vi "UiCharts_gm.vi"() -> ()   [LabVIEW 2011]
uses:
  Output - Cluster gas.ctl
  DBSqlSelectToArray(2DArrayString).vi
panel:
  in  "Tab Control":T1(tab)
  out "protocol":string[][](table)
  out "Temperaturregelung":cluster{"GM TS-2[°C]":dbl}(graph)
  in  "load":bool
  out "XY Graph":cluster{timestamp, dbl}[](graph)
  in  "end":timestamp=timestamp(3427221599.999 s since 1904-01-01) format="%<%X\n%x>T"
  in  "begin":timestamp=timestamp(3427135200 s since 1904-01-01) format="%<%X\n%x>T"
  in  "sensor":u16(ring) items=["DS1"=0, "TS4"=2, "TS5"=4, "pHS1"=6, "FS1"=8, "FS2"=10, "FS3"=12]
  in  "plant":u16(ring)=1 items=["B2G1", "B2G2", "GasMeas"]
  out "error out":errorcluster
  in  "stop":bool
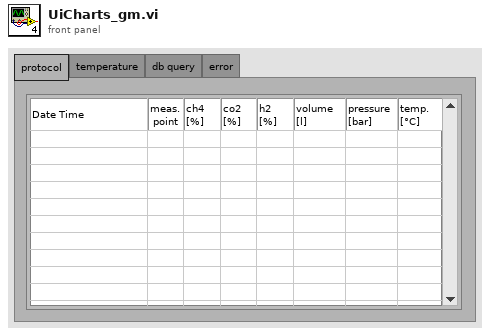
[diagram p1: front panel]
types:
  T1 = enum32{"protocol", "temperature", "db query", "error"}
  T2 = typedef "Output - Cluster gas.ctl" = cluster{"B2G2 MR V1.1 AUF":bool, "B2G2 MR V1.1 ZU":bool, "B2G2 MR V1 AUF":bool, "B2G2 MR V1 ZU":bool, "B2G1 T2 V1 AUF":bool, "B2G1 T2 V1 ZU":bool, "B2G1 T2 V1.1 AUF":bool, "B2G1 T2 V1.1 ZU":bool, "B2G2 T2 V1 AUF":bool, "B2G2 T2 V1 ZU":bool, "B2G2 T2 V1.1 ZU":bool, "B2G2 T2 V1.1 AUF":bool, "B2G1 MR V1 AUF":bool, "B2G1 MR V1 ZU":bool, "B2G1 MR V1.1 AUF":bool, "B2G1 MR V1.1 ZU":bool, "B2G1 HR V1 AUF":bool, "B2G1 HR V1 ZU":bool, "B2G1 HR V1.1 AUF":bool, "B2G1 HR V1.1 ZU":bool, "Fab1 HR V1 AUF":bool, "Fab1 HR V1 ZU":bool, "Fab1 HR V1.1 AUF":bool, "Fab1 HR V1.1 ZU":bool, "Fab1 MR V1 AUF":bool, "Fab1 MR V1 ZU":bool, "Fab1 MR V1.1 AUF":bool, "Fab1 MR V1.1 ZU":bool, "Fab1 BL V1 AUF":bool, "Fab1 BL V1 ZU":bool, "Fab1 BL V1.1 AUF":bool, "Fab1 BL V1.1 ZU":bool, "Fab2 HR V1 AUF":bool, "Fab2 HR V1 ZU":bool, "Fab2 HR V1.1 AUF":bool, "Fab2 HR V1.1 ZU":bool, "Fab2 MR V1 AUF":bool, "Fab2 MR V1 ZU":bool, "Fab2 MR V1.1 AUF":bool, "Fab2 MR V1.1 ZU":bool, "GA1 ch4 [%]":dbl, "GA1 co2 [%]":dbl, "GA1 h2 [%]":dbl, "GM P1 RUN":bool, "GM V-1 AUF":bool, "GM V-1 ZU":bool, "GM V-2 AUF":bool, "GM V-2 ZU":bool, "GM V-3 AUF":bool, "GM V-3 ZU":bool, "GM V-4 AUF":bool, "GM V-4 ZU":bool, "GM P2 RUN":bool, "GM GZ-1 [imp]":u32, "GM DS-2 [bar]":dbl, "GM DS-1 [bar]":dbl, "GM TS-1 [°C]":dbl, "GM TS-2[°C]":dbl, "gas_values":cluster{"timestamp":timestamp, "GM DS-2 [bar]":dbl, "GA1 ch4 [%]":dbl, "GA1 co2 [%]":dbl, "GA1 h2 [%]":dbl, "GM DS-1 [bar]":dbl, "GM TS-1 [°C]":dbl, "GM TS-2 [°C]":dbl, "GM GZ-1 [l]":dbl, "empty":bool, "measuring point":u8}, "measuring mode":u8}
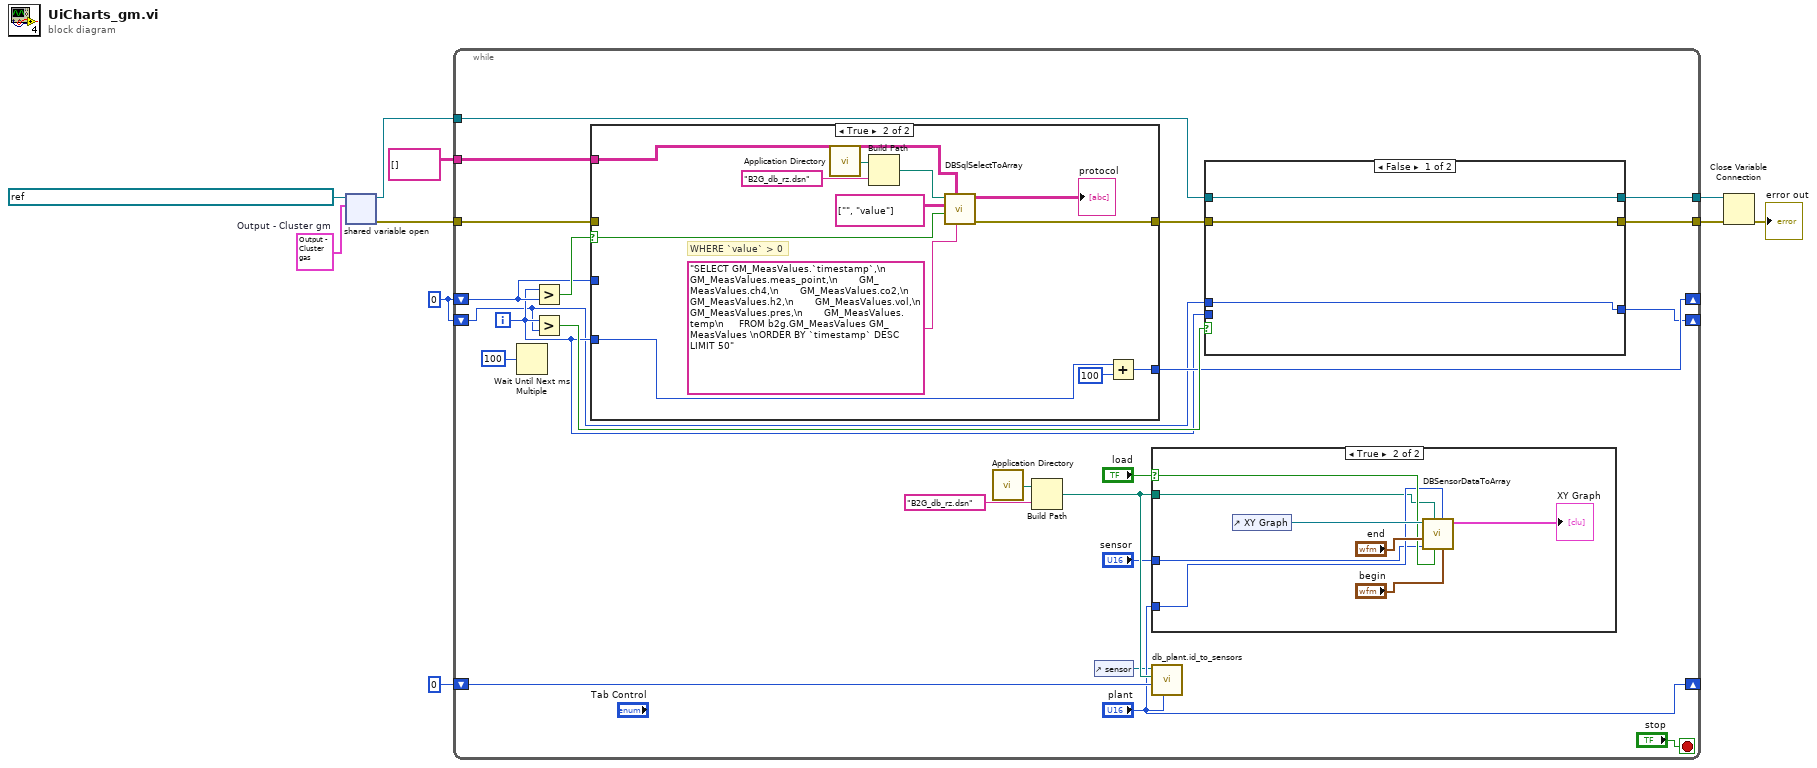
[diagram p0: block diagram]
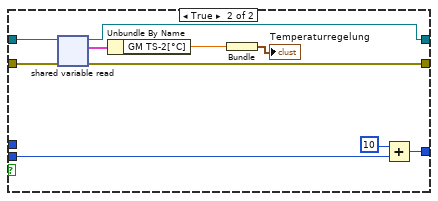
[diagram p4: hidden frame]
diagram:
  w9 = T2 {"B2G2 MR V1.1 AUF"=FALSE, "B2G2 MR V1.1 ZU"=FALSE, "B2G2 MR V1 AUF"=FALSE, "B2G2 MR V1 ZU"=FALSE, "B2G1 T2 V1 AUF"=FALSE, "B2G1 T2 V1 ZU"=FALSE, "B2G1 T2 V1.1 AUF"=FALSE, "B2G1 T2 V1.1 ZU"=FALSE, "B2G2 T2 V1 AUF"=FALSE, "B2G2 T2 V1 ZU"=FALSE, "B2G2 T2 V1.1 ZU"=FALSE, "B2G2 T2 V1.1 AUF"=FALSE, "B2G1 MR V1 AUF"=FALSE, "B2G1 MR V1 ZU"=FALSE, "B2G1 MR V1.1 AUF"=FALSE, "B2G1 MR V1.1 ZU"=FALSE, "B2G1 HR V1 AUF"=FALSE, "B2G1 HR V1 ZU"=FALSE, "B2G1 HR V1.1 AUF"=FALSE, "B2G1 HR V1.1 ZU"=FALSE, "Fab1 HR V1 AUF"=FALSE, "Fab1 HR V1 ZU"=FALSE, "Fab1 HR V1.1 AUF"=FALSE, "Fab1 HR V1.1 ZU"=FALSE, "Fab1 MR V1 AUF"=FALSE, "Fab1 MR V1 ZU"=FALSE, "Fab1 MR V1.1 AUF"=FALSE, "Fab1 MR V1.1 ZU"=FALSE, "Fab1 BL V1 AUF"=FALSE, "Fab1 BL V1 ZU"=FALSE, "Fab1 BL V1.1 AUF"=FALSE, "Fab1 BL V1.1 ZU"=FALSE, "Fab2 HR V1 AUF"=FALSE, "Fab2 HR V1 ZU"=FALSE, "Fab2 HR V1.1 AUF"=FALSE, "Fab2 HR V1.1 ZU"=FALSE, "Fab2 MR V1 AUF"=FALSE, "Fab2 MR V1 ZU"=FALSE, "Fab2 MR V1.1 AUF"=FALSE, "Fab2 MR V1.1 ZU"=FALSE, "GA1 ch4 [%]"=0.0, "GA1 co2 [%]"=0.0, "GA1 h2 [%]"=0.0, "GM P1 RUN"=FALSE, "GM V-1 AUF"=FALSE, "GM V-1 ZU"=FALSE, "GM V-2 AUF"=FALSE, "GM V-2 ZU"=FALSE, "GM V-3 AUF"=FALSE, "GM V-3 ZU"=FALSE, "GM V-4 AUF"=FALSE, "GM V-4 ZU"=FALSE, "GM P2 RUN"=FALSE, "GM GZ-1 [imp]"=0, "GM DS-2 [bar]"=0.0, "GM DS-1 [bar]"=0.0, "GM TS-1 [°C]"=0.0, "GM TS-2[°C]"=0.0, "gas_values"={"timestamp"=timestamp(0 s since 1904-01-01), "GM DS-2 [bar]"=0.0, "GA1 ch4 [%]"=0.0, "GA1 co2 [%]"=0.0, "GA1 h2 [%]"=0.0, "GM DS-1 [bar]"=0.0, "GM TS-1 [°C]"=0.0, "GM TS-2 [°C]"=0.0, "GM GZ-1 [l]"=0.0, "empty"=FALSE, "measuring point"=0}, "measuring mode"=0}  # Output - Cluster gm
  w5 = i64 0
  n1 = shared-variable-open(refnum<k21> "ni.var.psp://10.27.40.21/variables - gas/data - network - gas" ("Output Var"), w9) -> (w8:refnum<k21>, w1:errorcluster)  [unwired: 2 in]
  n2 = while {
    tunnel: w8 -> [w33]
    tunnel: [w32] -> w7
    tunnel: string[][] [] ("data") -> [w31]
    shift-right: [w27] -> _
    shift-left: w5 -> [w28]
    shift-right: [w26] -> _
    shift-left: w5 -> [w23]
    tunnel: w1 -> [w19]
    tunnel: [w18] -> w4
    shift-right: ["plant"] -> _
    shift-left: u16 0 ("plant") -> [w17]
    i -> [w24]
    stop <- "stop" stop-if-true
    n3 = Wait Until Next ms Multiple(millisecond multiple=100) -> ()  [unwired: 1 out]
    n4 = Greater?(x=w24, y=w28) -> (0:w30:bool)
    n5 = Greater?(x=w24, y=w23) -> (0:w29:bool)
    n6 = case shown="True" w30 {
      selector: w30 -> [_ w45]
      tunnel: [w43 w54] -> w27
      tunnel: w28 -> [w43 _]
      tunnel: w24 -> [_ w55]
      tunnel: w31 -> [_ w48]
      tunnel: [w42 w47] -> w21
      tunnel: w19 -> [w42 _]
      frame False {
      }
      frame True {
        # "WHERE `value` > 0"
        n7 = call <vilib>:"Application Directory.vi"() -> ("Application Directory"=w50:path)
        n8 = Build Path(base path=w50, name or relative path="B2G_db_rz.dsn" ("Name of ini file 2")) -> (appended path=w49:path)
        n9 = call-poly "DBSqlSelectToArray.vi"("String"="SELECT GM_MeasValues.`timestamp`,\n       GM_MeasValues.meas_point,\n       GM_MeasValues.ch4,\n       GM_MeasValues.co2,\n       GM_MeasValues.h2,\n       GM_MeasValues.vol,\n       GM_MeasValues.pres,\n       GM_MeasValues.temp\n     FROM b2g.GM_MeasValues GM_MeasValues \nORDER BY `timestamp` DESC LIMIT 50" ("SQL query"), "shift reg in"=w48, "enable"=w45, "format"=string[][] [["", "value"]] ("columns"), "connection information"=w49) -> ("error out"=w47:errorcluster, "shift reg out"=→"protocol":string[][])  [unwired: 5 in]
        n10 = Add(x=w55, y=i64 100) -> (x+y=w54:i64)
      }
    }
    n11 = call <vilib>:"Application Directory.vi"() -> ("Application Directory"=w16:path)
    n12 = Build Path(base path=w16, name or relative path="B2G_db_rz.dsn" ("Name of ini file 2")) -> (appended path=w14:path)
    n13 = control-ref of="sensor"() -> (w11:refnum<vi>)
    n14 = case shown="True" "load" {
      selector: "load" -> [_ w37]
      tunnel: "plant" -> [_ w36]
      tunnel: w14 -> [_ w35]
      tunnel: "sensor" -> [_ w34]
      frame False {
      }
      frame True {
        n15 = control-ref of="XY Graph"() -> (w39:refnum<vi>)
        n16 = call "DBSensorDataToArray.vi"("begin"="begin", "plant"=w36, "load"=w37, "appended path"=w35, "sensor"=w34, "end"="end", "XYGraph in"=w39) -> ("shift reg out"=→"XY Graph":cluster{timestamp, dbl}[])  [unwired: 3 in, 1 out]
      }
    }
    n17 = call "db_plant.id_to_sensors.vi"("plant"="plant", "shift reg"=w17, "db path"=w14, "Ring in"=w11) -> ()  [unwired: 8 in]
    n18 = case shown="False" w29 {
      tunnel: w33 -> [w57 w68]
      tunnel: [w57 w67] -> w32
      tunnel: [w58 w64] -> w26
      tunnel: w24 -> [_ w63]
      tunnel: w23 -> [w58 _]
      tunnel: w21 -> [w56 w62]
      tunnel: [w56 w61] -> w18
      frame False {
      }
      frame True {
        n19 = shared-variable-read(w68, w62) -> (w67:refnum<k21>, w61:errorcluster, w66:T2)  [unwired: 1 out]
        n20 = Unbundle By Name(w66) -> ("GM TS-2[°C]"=w60:dbl)
        n21 = Bundle("GM TS-2[°C]"=w60) -> (→"Temperaturregelung":cluster{"GM TS-2[°C]":dbl})  [unwired: 1 in]
        n22 = Add(x=10, y=w63) -> (x+y=w64:i32)
      }
    }
  }
  n23 = Close Variable Connection(8:w4, 11:w7) -> (0:→"error out":errorcluster)
